vi "SPADQ_SetInputImpedance.vi"(5 "channel":u32, 7 "mode":u32, 8 "error in (no error)":errorcluster, 9 "adq_num":i32, 10 "adq_cu_ptr in":refnum<k24>, 11 "ADQAPI Ref":refnum<k24>) -> (0 "error out":errorcluster, 3 "ADQAPI Ref (out)":refnum<k24>)   [LabVIEW 2022 SP3]
doc: "DLL_IMPORT int ADQ_SetInputImpedance(void* adq_cu_ptr, int adq_num , unsigned int channel, unsigned int mode);"
uses:
  C:/Windows/System32/ADQAPI_dotNet_helper.dll
panel:
  out "ADQ_SetInputImpedance":i32
  # "Not for use with ADQ7!!!!!!!!!!!!!!!!!!!!!!!!!!"
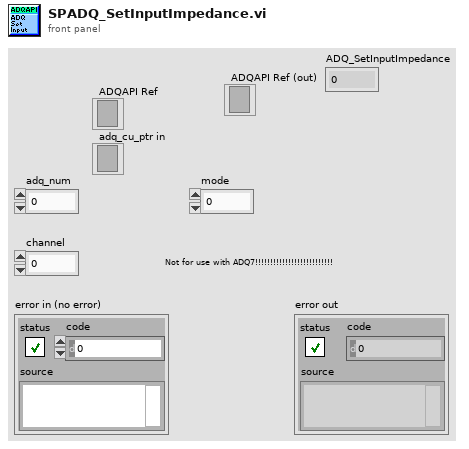
[diagram p1: front panel]
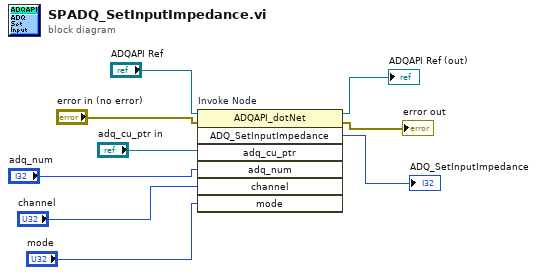
[diagram p0: block diagram]
diagram:
  n1 = invoke on="Invoke Node" class="ADQAPI_dotNet" method="ADQ_SetInputImpedance"(reference="ADQAPI Ref", error in="error in (no error)", "adq_cu_ptr"="adq_cu_ptr in", "adq_num"="adq_num", "channel"="channel", "mode"="mode") -> (reference out=→"ADQAPI Ref (out)":refnum<k24>, error out=→"error out":errorcluster, "ADQ_SetInputImpedance"=→"ADQ_SetInputImpedance":i32)  [unwired: 1 in, 4 out]
